vi "scp_file_transfer.vi"(0 "File transfer 2":T1, 11 "error in (no error)":errorcluster) -> (4 "file status":bool, 6 "File transfer 3":T1, 15 "error out":errorcluster)   [LabVIEW 2022 SP3]
uses:
  <vilib>/net/SSH/Client/OpenSSH/OpenSSH Client.lvclass
  C:/Program Files (x86)/National Instruments/LabVIEW 2022/vi.lib/net/SSH/Client/Generic/Generic Client.lvclass
  <vilib>/net/SFTP/API/Upload File.vi
  <vilib>/net/SFTP/Session/Session.lvclass
  <vilib>/net/SFTP/NI_SFTP.lvlib
  <vilib>/net/SFTP/Connect (OpenSSH).vi
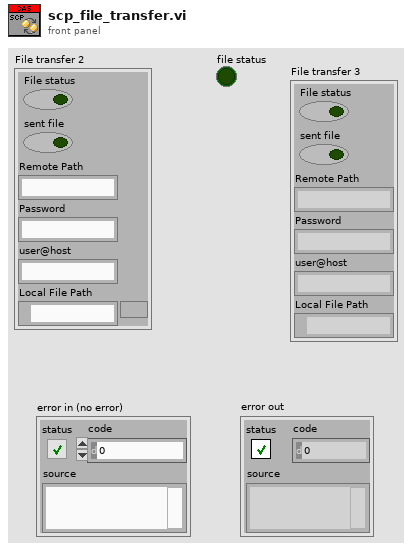
[diagram p1: front panel]
types:
  T1 = cluster{"File status":bool, "sent file":bool, "Remote Path":string, "Password":string, "user@host":string, "Local File Path":path}
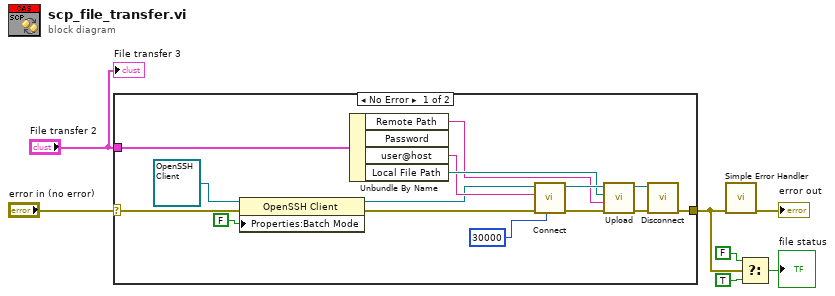
[diagram p0: block diagram]
diagram:
  n1 = case shown="No Error" "error in (no error)" {
    selector: "error in (no error)" -> [w18 w23]
    tunnel: [w16 w23] -> w2
    tunnel: "File transfer 2" -> [w14 _]
    frame No Error {
      n2 = property class="OpenSSH Client"(reference=refnum<class "OpenSSH Client.lvclass"> refnum ("NI_SSH.lvlib:OpenSSH Client"), error in=w18, "Properties:Batch Mode"=FALSE ("Batch Mode")) -> (reference out=w8:refnum<class "OpenSSH Client.lvclass">, error out=w22:errorcluster)
      n3 = Unbundle By Name(w14) -> ("Remote Path"=w12:string, "user@host"=w10:string, "Local File Path"=w13:path)  [unwired: 1 out]
      n4 = call-poly <vilib>:"Connect.vi"("timeout (ms)"=30000, "error in"=w22, "user@host"=w10, "client"=w8) -> ("error out"=w20:errorcluster, "session"=w21:refnum<class "Session.lvclass">)  [unwired: 6 in]
      n5 = call-poly <vilib>:"Upload.vi"("error in"=w20, "remote path"=w12, "local path"=w13, "session in"=w21) -> ("error out"=w17:errorcluster, "session out"=w15:refnum<class "Session.lvclass">)  [unwired: 6 in]
      n6 = call-dynamic "Disconnect.vi"("error in"=w17, "session in"=w15) -> ("error out"=w16:errorcluster)  [unwired: 6 in, 3 out]
    }
    frame Error {
    }
  }
  n7 = call <vilib>:"Simple Error Handler.vi"("error in (no error)"=w2) -> ("error out"=→"error out":errorcluster)  [unwired: 4 in, 4 out]
  n8 = Select(t=FALSE, s=w2, f=TRUE) -> (s? t:f=→"file status":bool)
  "File transfer 3" <- "File transfer 2"
